vi "AddEllement (SubVI).vi"() -> (3 "1D Array 5":string[](array[string]))   [LabVIEW 2017]
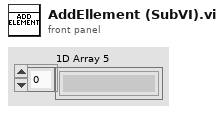
[diagram p1: front panel]
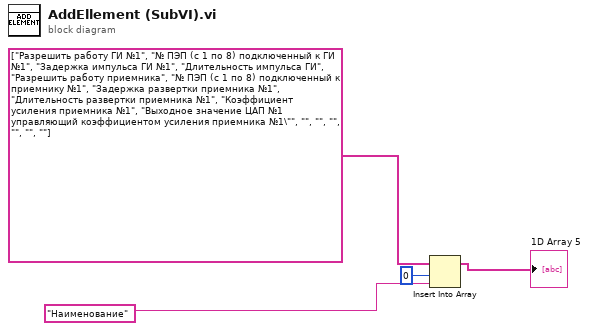
[diagram p0: block diagram]
diagram:
  n1 = Insert Into Array(array=string[] ["Разрешить работу ГИ №1", "№ ПЭП (с 1 по 8) подключенный к ГИ №1", "Задержка импульса ГИ №1", "Длительность импульса ГИ", "Разрешить работу приемника", "№ ПЭП (с 1 по 8) подключенный к приемнику №1", "Задержка развертки приемника №1", "Длительность развертки приемника №1", "Коэффициент усиления приемника №1", "Выходное значение ЦАП №1 управляющий коэффициентом усиления приемника №1\"", "", "", "", "", "", ""] ("1D Array 5"), index=0, new element="Наименование" ("new element/subarray")) -> (→"1D Array 5":string[])
